vi "RunCopyYesterday.vi"() -> ()   [LabVIEW 2012]
uses:
  <vilib>/Utility/file.llb/Read From Spreadsheet File (string).vi
panel:
  out "OK 2":bool
  out "OK":bool
  out "OK 3":bool
  out "Numeric":i32
  out "all rows":string[][](array[string])
  out "element":string
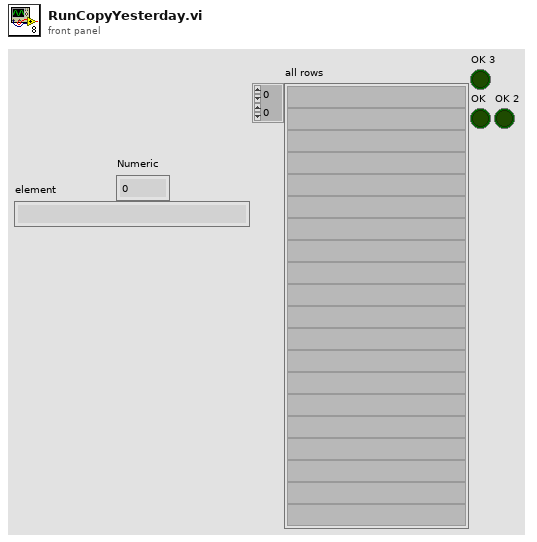
[diagram p1: front panel]
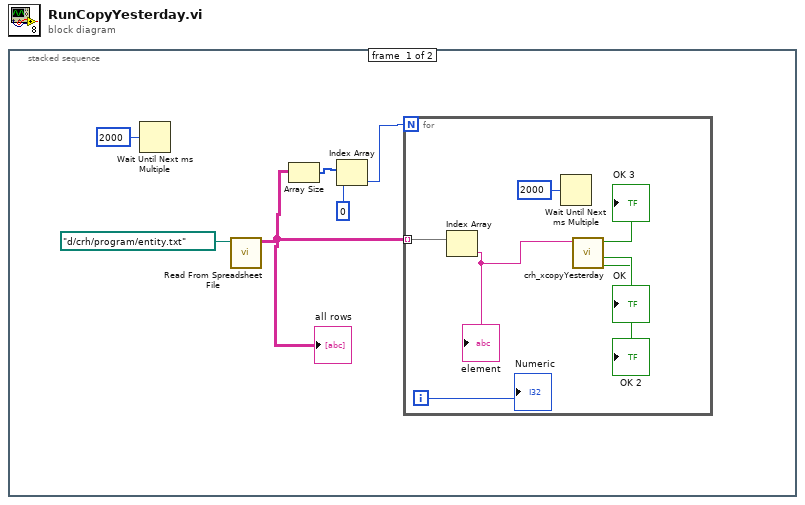
[diagram p0: block diagram]
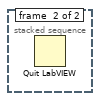
[diagram p2: hidden frame]
diagram:
  n1 = stacked-sequence {
    frame #0 {
      n2 = Wait Until Next ms Multiple(millisecond multiple=u32 2000) -> ()  [unwired: 1 out]
      n3 = call-poly <vilib>:"Read From Spreadsheet File.vi"("file path (dialog if empty)"=path "d:/crh/program/entity.txt") -> ("all rows"=w4:string[][])  [unwired: 6 in, 4 out]
      "all rows" <- w4
      n4 = Array Size(array=w4) -> (size(s)=w6:i32[])
      n5 = Index Array(array=w6, index=0) -> (element=w2:i32)
      n6 = for {
        N: w2 -> [_]
        tunnel: w4 -> [w13] mode=indexing
        i -> [w11]
        n7 = Index Array(array=w13) -> (element=w12:string)  [unwired: 1 in]
        "element" <- w12
        n8 = Wait Until Next ms Multiple(millisecond multiple=u32 2000) -> ()  [unwired: 1 out]
        n9 = call "crh_xcopyYesterday.vi"("folder"=w12) -> ("OK 2"=→"OK 2":bool, "OK"=→"OK":bool, "OK 3"=→"OK 3":bool)  [unwired: 8 in]
        "Numeric" <- w11
      }
    }
    frame #1 {
      n10 = Quit LabVIEW() -> ()  [unwired: 1 in]
    }
  }
